vi "addcommadouble.vi"(10 "input":dbl) -> (2 "output":string)   [LabVIEW 2012]
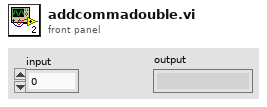
[diagram p1: front panel]
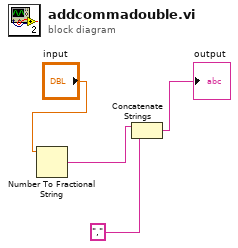
[diagram p0: block diagram]
diagram:
  n1 = Number To Fractional String(number="input") -> (F-format string=w3:string)  [unwired: 3 in]
  n2 = Concatenate Strings(w3, ",") -> (→"output":string)
